vi "Atualiza_array_prioridade.vi"() -> (0 "error out":errorcluster, 3 "refnum":T1)   [LabVIEW 2019]
uses:
  <vilib>/Utility/config.llb/Config Data RefNum.ctl
  <vilib>/Utility/config.llb/Write Key (Boolean).vi
  <vilib>/Utility/config.llb/NI_LVConfig.lvlib
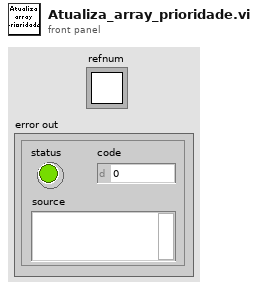
[diagram p1: front panel]
types:
  T1 = typedef "NI_LVConfig.lvlib/Config Data RefNum.ctl" = refnum<k1>
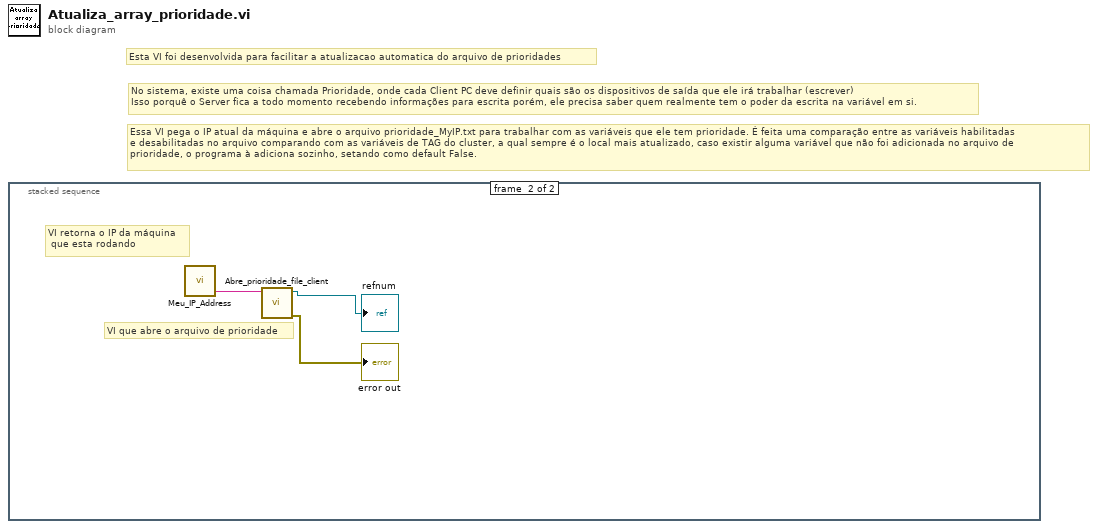
[diagram p0: block diagram]
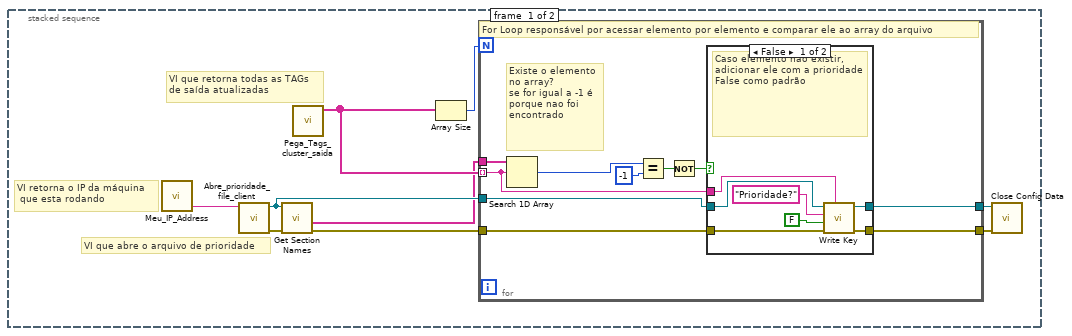
[diagram p2: hidden frame]
diagram:
  # "Essa VI pega o IP atual da máquina e abre o arquivo prioridade_MyIP.txt para trabalhar com as variáveis que ele tem prioridade. É feita uma comparação entre as variáveis habilitadas\ne desabilitadas no arquivo comparando com as variáveis de TAG do cluster, a qual sempre é o local mais atualizado, caso existir alguma variável que não foi adicionada no arquivo de \nprioridade, o programa à adiciona sozinho, setando como default False."
  # "No sistema, existe uma coisa chamada Prioridade, onde cada Client PC deve definir quais são os dispositivos de saída que ele irá trabalhar (escrever)\nIsso porquê o Server fica a todo momento recebendo informações para escrita porém, ele precisa saber quem realmente tem o poder da escrita na variável em si."
  # "Esta VI foi desenvolvida para facilitar a atualizacao automatica do arquivo de prioridades"
  n1 = stacked-sequence {
    frame #0 {
      # "VI que abre o arquivo de prioridade"
      # "VI retorna o IP da máquina\n que esta rodando"
      # "VI que retorna todas as TAGs \nde saída atualizadas"
      n2 = call "Meu_IP_Address.vi"() -> ("Meu IP"=w4:string)  [unwired: 4 in, 1 out]
      n3 = call "Abre_prioridade_file_client.vi"("Meu_Ip"=w4) -> ("error out"=w6:errorcluster, "refnum"=w5:T1)  [unwired: 9 in]
      n4 = call <vilib>:"Get Section Names.vi"("error in (no error)"=w6, "refnum"=w5) -> ("error out"=w3:errorcluster, "section names"=w1:string[])  [unwired: 7 in, 1 out]
      n5 = call "Pega_Tags_cluster_saida.vi"() -> ("Array Tags"=w7:string[])  [unwired: 10 in, 1 out]
      n6 = Array Size(array=w7) -> (size(s)=w2:i32)
      n7 = for {
        N: w2 -> [_]
        tunnel: w7 -> [w19] mode=indexing
        tunnel: w1 -> [w18]
        tunnel: w3 -> [w12]
        tunnel: w5 -> [w17]
        tunnel: [w11] -> w9
        tunnel: [w10] -> w8
        # "Existe o elemento\nno array?\nse for igual a -1 é porque nao foi encontrado"
        # "For Loop responsável por acessar elemento por elemento e comparar ele ao array do arquivo"
        n8 = Search 1D Array(1D array=w18, element=w19) -> (index of element=w14:i32)  [unwired: 1 in]
        n9 = Equal?(x=w14, y=-1) -> (x = y?=w16:bool)
        n10 = Not(x=w16) -> (.not. x?=w13:bool)
        n11 = case shown="False" w13 {
          tunnel: w19 -> [w26 _]
          tunnel: w17 -> [w25 w27]
          tunnel: w12 -> [w23 w28]
          tunnel: [w21 w28] -> w11
          tunnel: [w20 w27] -> w10
          frame False {
            # "Caso elemento não existir, adicionar ele com a prioridade False como padrão"
            n12 = call-poly <vilib>:"Write Key.vi"("section"=w26, "error in (no error)"=w23, "value"=FALSE, "key"="Prioridade?", "refnum"=w25) -> ("error out"=w21:errorcluster, "refnum out"=w20:T1)  [unwired: 4 in, 1 out]
          }
          frame True {
            # "Caso o elemento já existir no arquivo de pioridade, não fazer nada"
          }
        }
      }
      n13 = call <vilib>:"Close Config Data.vi"("error in (no error)"=w9, "refnum"=w8) -> ()  [unwired: 8 in, 2 out]
    }
    frame #1 {
      # "VI que abre o arquivo de prioridade"
      # "VI retorna o IP da máquina\n que esta rodando"
      n14 = call "Meu_IP_Address.vi"() -> ("Meu IP"=w31:string)  [unwired: 4 in, 1 out]
      n15 = call "Abre_prioridade_file_client.vi"("Meu_Ip"=w31) -> ("error out"=→"error out":errorcluster, "refnum"=→"refnum":T1)  [unwired: 9 in]
    }
  }
